vi "Pfeiffer-RVC300.remove services.vi"(0 "i ref in":refnum<vi>, 3 "ms timeout (10000)":i32=10000, 5 "error in (no error)":errorcluster) -> (14 "i ref out":refnum<vi>, 17 "timed out":bool, 19 "error out":errorcluster)   [LabVIEW 2014, in "Pfeiffer-RVC300.lvlib"]
doc: "Removes my DIM services."
uses:
  Pfeiffer-RVC300.lvlib
  CSlibraries-extern/DimLVEvent/LVDimInterface/LVDimInterface.lvlib
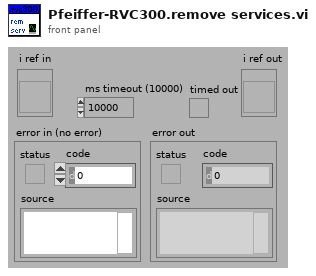
[diagram p1: front panel]
types:
  T1 = typedef "Pfeiffer-RVC300.lvlib/Pfeiffer-RVC300.i attribute.ctl" = cluster{"interfaceInitialized":bool, "VISAResource":refnum<visa-resource-name>, "WaitingTime":u32, "nomValues":T2, "actValues":T2}
  T2 = typedef "Pfeiffer-RVC300.lvlib/Pfeiffer-RVC300.parameters.ctl" = cluster{"regulationMode":T3, "valveType":string, "sensorType":string, "valveState":string, "flow":dbl, "pressure":dbl, "serviceIDs":cluster{"regulationModeID":i32, "valveTypeID":i32, "sensorTypeID":i32, "valveStateID":i32, "flowID":i32, "pressureID":i32}}
  T3 = typedef "Pfeiffer-RVC300.lvlib/Pfeiffer-RVC300.regulation mode.ctl" = enum16{"unknown", "Pressure", "Flow", "Wait"}
  T4 = cluster{"regulationModeID":i32, "valveTypeID":i32, "sensorTypeID":i32, "valveStateID":i32, "flowID":i32, "pressureID":i32}
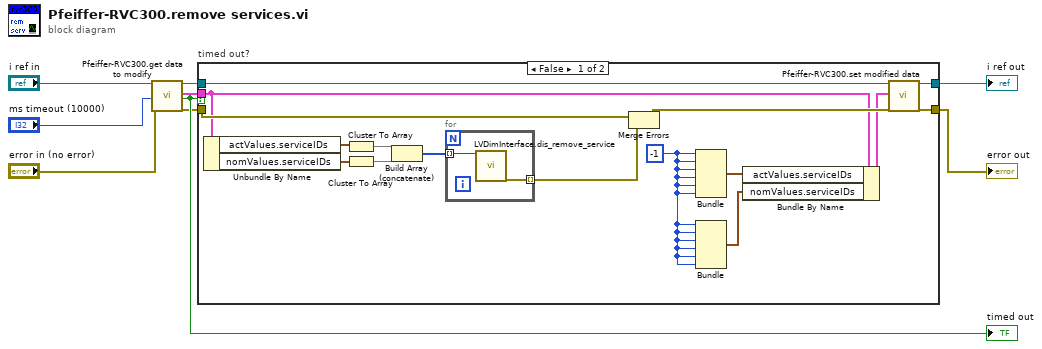
[diagram p0: block diagram]
diagram:
  n1 = call "Pfeiffer-RVC300.get data to modify.vi"("i ref in"="i ref in", "ms timeout (10000)"="ms timeout (10000)", "error in (no error)"="error in (no error)") -> ("i ref out"=w3:refnum<vi>, "i attribute"=w1:T1, "timed out"=w4:bool, "error out"=w2:errorcluster)  [unwired: 13 in]
  "timed out" <- w4
  n2 = case "timed out?" shown="False" w4 {
    tunnel: w3 -> [w20 w29]
    tunnel: [w25 w29] -> w6
    tunnel: w2 -> [w23 w28]
    tunnel: [w24 w28] -> w8
    tunnel: w1 -> [w19 _]
    frame False {
      w13 = -1
      n3 = Unbundle By Name(w19) -> ("actValues.serviceIDs"=w11:T4, "nomValues.serviceIDs"=w10:T4)
      n4 = Cluster To Array(cluster=w11) -> (array=w18:i32[])
      n5 = Cluster To Array(cluster=w10) -> (array=w17:i32[])
      n6 = Build Array (concatenate)(w18, w17) -> (w15:i32[])
      n7 = for {
        tunnel: w15 -> [w27] mode=indexing
        tunnel: [w26] -> w14 mode=indexing
        n8 = call "LVDimInterface.dis_remove_service.vi"("my_serviceID"=w27) -> ("error out"=w26:errorcluster)  [unwired: 18 in]
      }
      n9 = Merge Errors(w23, w14) -> (w22:errorcluster)
      n10 = Bundle(w13, w13, w13, w13, w13, w13) -> (w16:cluster{i32, i32, i32, i32, i32, i32})  [unwired: 1 in]
      n11 = Bundle(w13, w13, w13, w13, w13, w13) -> (w12:cluster{i32, i32, i32, i32, i32, i32})  [unwired: 1 in]
      n12 = Bundle By Name(cluster=w19, "actValues.serviceIDs"=w16, "nomValues.serviceIDs"=w12) -> (w21:T1)
      n13 = call "Pfeiffer-RVC300.set modified data.vi"("i ref in"=w20, "i attribute"=w21, "error in (no error)"=w22) -> ("i ref out"=w25:refnum<vi>, "error out"=w24:errorcluster)  [unwired: 15 in]
    }
    frame True {
    }
  }
  "error out" <- w8
  "i ref out" <- w6
